vi "Run Test Case.vi"(8 "error in (no error)":errorcluster, 10 "Test Case":refnum<class "LUnit Test Case.lvclass">, 11 "Execution API In":refnum<class "Execution API.lvclass">) -> (0 "error out":errorcluster, 3 "Execution API Out":refnum<class "Execution API.lvclass">)   [LabVIEW 2020, in "Execution API.lvclass"]
doc: "Run a single test case."
uses:
  Execution API.lvclass
  LUnit Test Case.lvclass
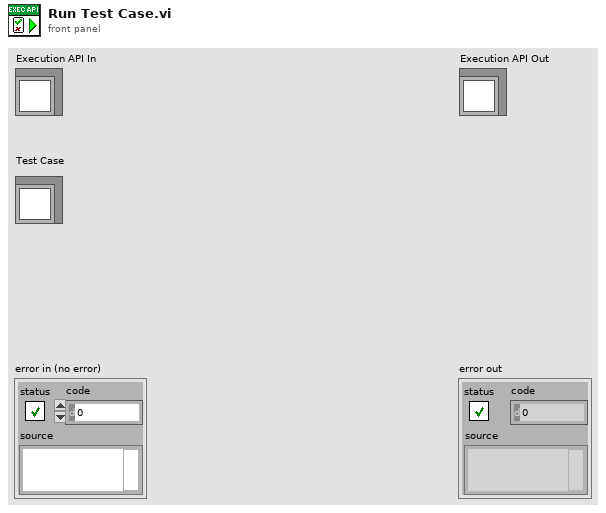
[diagram p1: front panel]
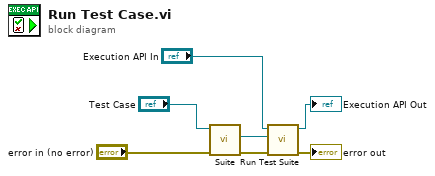
[diagram p0: block diagram]
diagram:
  n1 = call-dynamic "Suite.vi"("error in (no error)"="error in (no error)", "LUnit Test Case In"="Test Case") -> ("error out"=w3:errorcluster, "LUnit Test Suite Out"=w4:refnum<class "LUnit Test Suite.lvclass">)  [unwired: 7 in, 1 out]
  n2 = call "Run Test Suite.vi"("error in (no error)"=w3, "Test Suite"=w4, "Execution API In"="Execution API In") -> ("error out"=→"error out":errorcluster, "Execution API Out"=→"Execution API Out":refnum<class "Execution API.lvclass">)  [unwired: 7 in]
